vi "Test Controller.vi"() -> ()   [LabVIEW 2014]
uses:
  Ctrls/Translation Stage Cluster.ctl
  C:/Projects/Serial Sectioning OCT/Software/Thorlabs.MotionControl.Controls.dll
  Thorlabs.MotionControl.Controls.dll
panel:
  out "GetMoveAbsolutePosition":dbl
  in  "Position":dbl format="%#_13g"
  in  "Move":bool
  out "error out":errorcluster
  in  "Stop Button":bool
  in  "SerialNumber":string="45876060"
  in  "LTS Reference":refnum<k24>(container)
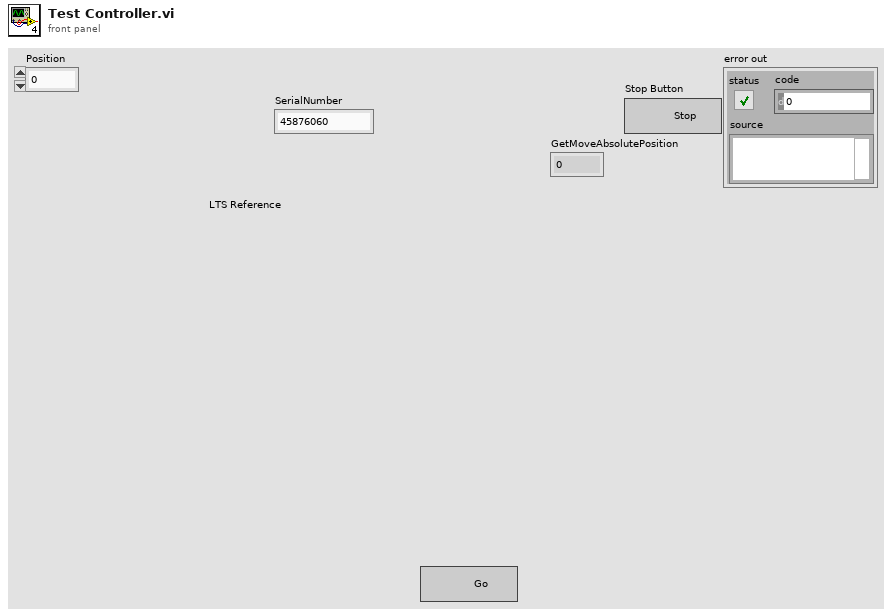
[diagram p1: front panel]
types:
  T1 = typedef "Translation Stage Cluster.ctl" = cluster{"Device SN":string, "Is.Connected?":bool, "Is.Enabled?":bool, "Position":dbl, "AccelerationMaximum":dbl, "VelocityMaximum":dbl, "Acceleration":dbl, "Velocity":dbl, "waitTimeout (ms)":i32}
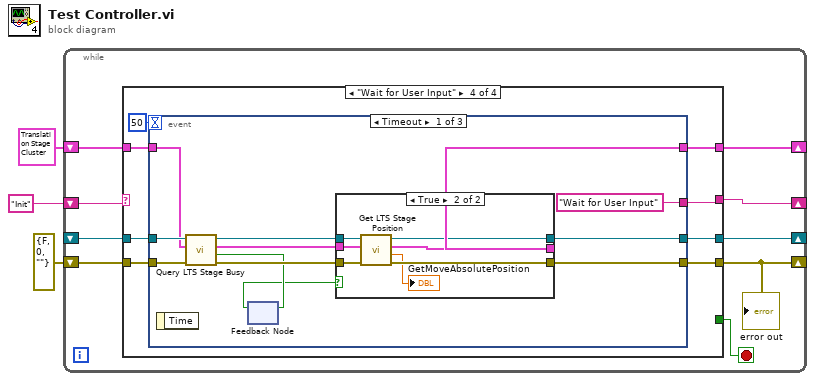
[diagram p0: block diagram]
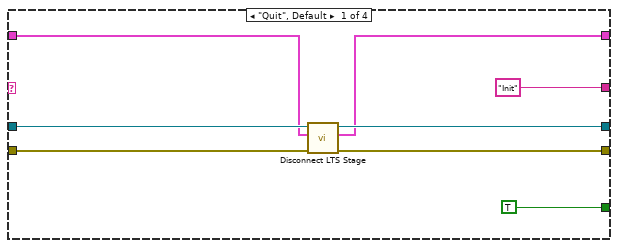
[diagram p2: hidden frame]
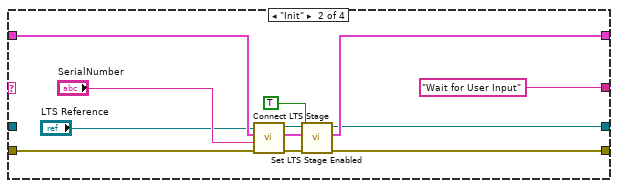
[diagram p3: hidden frame]
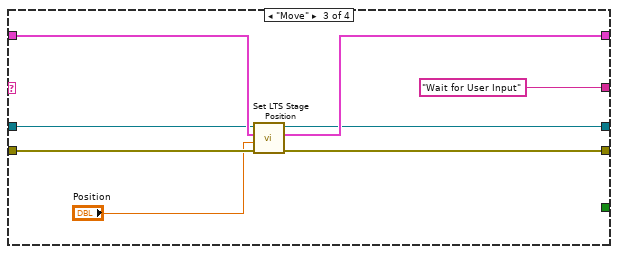
[diagram p4: hidden frame]
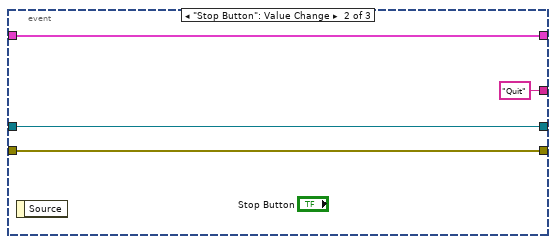
[diagram p6: hidden frame]
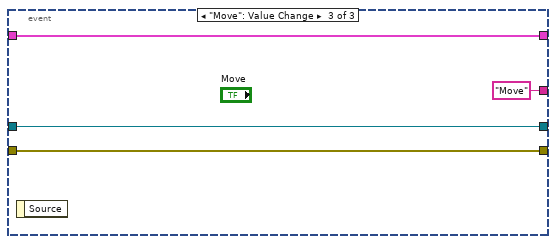
[diagram p7: hidden frame]
diagram:
  n1 = while {
    shift-right: [w11] -> _
    shift-left: "Init" -> [w12]
    shift-right: [w9] -> _
    shift-left: T1 {"Device SN"="45876539", "Is.Connected?"=FALSE, "Is.Enabled?"=FALSE, "Position"=0.0, "AccelerationMaximum"=0.0, "VelocityMaximum"=0.0, "Acceleration"=0.0, "Velocity"=0.0, "waitTimeout (ms)"=0} ("Cluster out") -> [w8]
    shift-right: [w7] -> _
    shift-left: errorcluster {"status"=FALSE, "code"=0, "source"=""} ("error out") -> [w6]
    shift-right: [w4] -> _
    shift-left: _ -> [w5]
    stop <- w10 stop-if-true
    n2 = case shown="\"Wait for User Input\"" w12 {
      tunnel: ["Init" "Wait for User Input" "Wait for User Input" w44] -> w11
      tunnel: [TRUE _ _ _] -> w10
      tunnel: [w13 w28 w34 w43] -> w9
      tunnel: w8 -> [w14 w27 w40 w42]
      tunnel: [w15 w25 w35 w48] -> w7
      tunnel: w6 -> [w16 w24 w39 w47]
      tunnel: w5 -> [w18 _ w37 w45]
      tunnel: [w17 w23 w33 w46] -> w4
      frame "Quit", Default {
        n3 = call "Disconnect LTS Stage.vi"("error in (no error)"=w16, "Cluster in"=w14, "LTS Reference In"=w18) -> ("error out"=w15:errorcluster, "Cluster out"=w13:T1, "LTS Reference Out"=w17:refnum<k24>)  [unwired: 6 in]
      }
      frame "Init" {
        n4 = call "Connect LTS Stage.vi"("error in (no error)"=w24, "SerialNumber"="SerialNumber", "Cluster in"=w27, "LTS Reference In"="LTS Reference") -> ("error out"=w32:errorcluster, "Cluster out"=w30:T1, "LTS Reference Out"=w31:refnum<k24>)  [unwired: 4 in, 1 out]
        n5 = call "Set LTS Stage Enabled.vi"("error in (no error)"=w32, "Enable?"=TRUE, "Cluster in"=w30, "LTS Reference In"=w31) -> ("error out"=w25:errorcluster, "Cluster out"=w28:T1, "LTS Reference Out"=w23:refnum<k24>)  [unwired: 5 in]
      }
      frame "Move" {
        n6 = call "Set LTS Stage Position.vi"("error in (no error)"=w39, "Position"="Position", "Cluster in"=w40, "LTS Reference In"=w37) -> ("error out"=w35:errorcluster, "Cluster out"=w34:T1, "LTS Reference Out"=w33:refnum<k24>)  [unwired: 5 in]
      }
      frame "Wait for User Input" {
        n7 = event shown="[0] Timeout" {
          selector: _ -> [_ _ _]
          dyn-events: _ -> [_ _ _]
          timeout: 50 -> [_ _ _]
          tunnel: [w55 w74 w78] -> w48
          tunnel: w47 -> [w60 w74 w78]
          tunnel: [w53 w73 w77] -> w46
          tunnel: w45 -> [w58 w73 w77]
          tunnel: ["Wait for User Input" "Quit" "Move"] -> w44
          tunnel: [w50 w72 w76] -> w43
          tunnel: w42 -> [w57 w72 w76]
          event Timeout {
            n8 = event-data() -> ()  [unwired: 1 in, 1 out]
            n9 = call "Query LTS Stage Busy.vi"("error in (no error)"=w60, "Cluster in"=w57, "LTS Reference In"=w58) -> ("error out"=w56:errorcluster, "IsDeviceBusy"=w52:bool, "Cluster out"=w51:T1, "LTS Reference Out"=w54:refnum<k24>)  [unwired: 5 in]
            n10 = feedback-in #1(w52) -> ()
            n11 = feedback #1() -> (w49:bool)  [unwired: 1 in]
            n12 = case shown="True" w49 {
              tunnel: w56 -> [w61 w70]
              tunnel: [w61 w69] -> w55
              tunnel: w54 -> [w63 w68]
              tunnel: [w63 w67] -> w53
              tunnel: w51 -> [w62 w66]
              tunnel: [w62 w65] -> w50
              frame False {
              }
              frame True {
                n13 = call "Get LTS Stage Position.vi"("error in (no error)"=w70, "Cluster in"=w66, "LTS Reference In"=w68) -> ("error out"=w69:errorcluster, "GetMoveAbsolutePosition"=→"GetMoveAbsolutePosition":dbl, "Cluster out"=w65:T1, "LTS Reference Out"=w67:refnum<k24>)  [unwired: 5 in]
              }
            }
          }
          event "Stop Button": Value Change {
            n14 = event-data() -> ()  [unwired: 1 in, 1 out]
          }
          event "Move": Value Change {
            n15 = event-data() -> ()  [unwired: 1 in, 1 out]
          }
        }
      }
    }
    "error out" <- w7
  }
